vi "LINC Parser.vi"(8 "error in (no error)":errorcluster, 10 "command in":string) -> (0 "error out":errorcluster, 2 "command":string, 4 "command arguments":string[][](array[string]))   [LabVIEW 2018, in "STEPkgDriver_LINC.lvlib"]
doc: "Parses the string command to separate the command from the arguments. Provides syntax checking to ensure it follows the \"<CMD> WITH | TO<argument 1>,<argument 2>, etc\" syntax."
uses:
  STEPkgDriver_LINC.lvlib
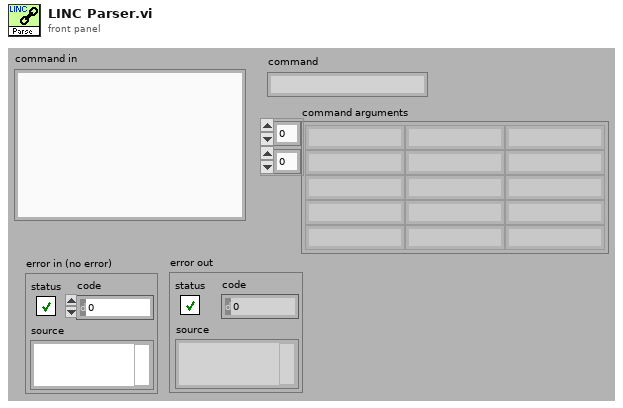
[diagram p1: front panel]
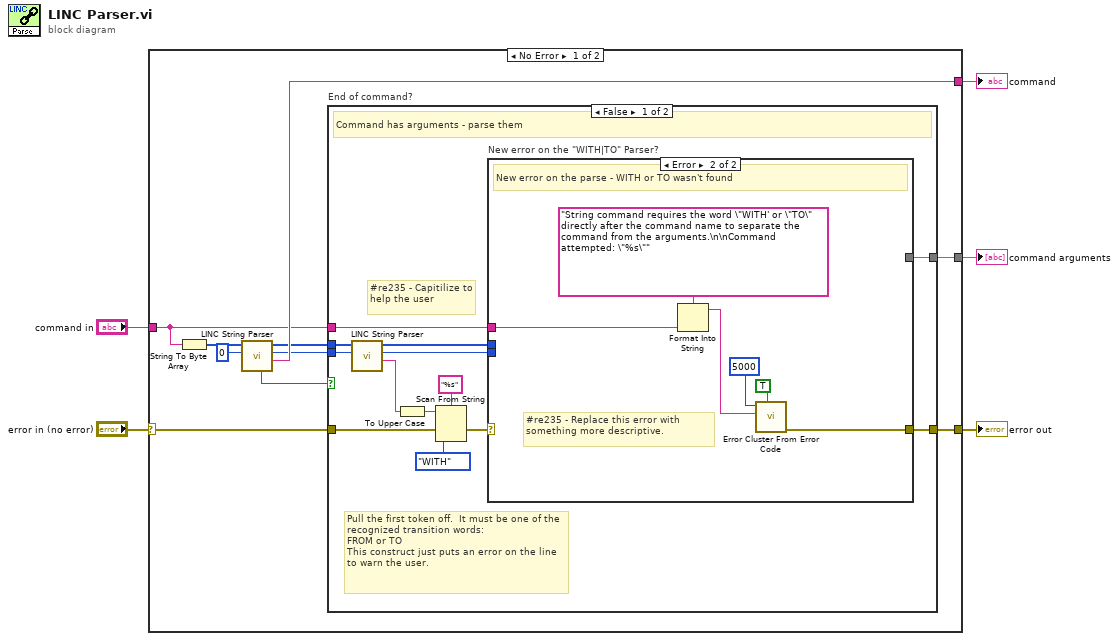
[diagram p0: block diagram]
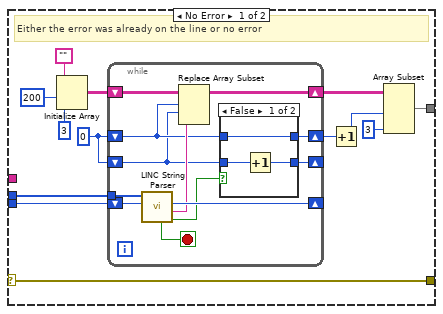
[diagram p2: hidden frame]
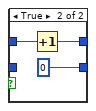
[diagram p3: hidden frame]
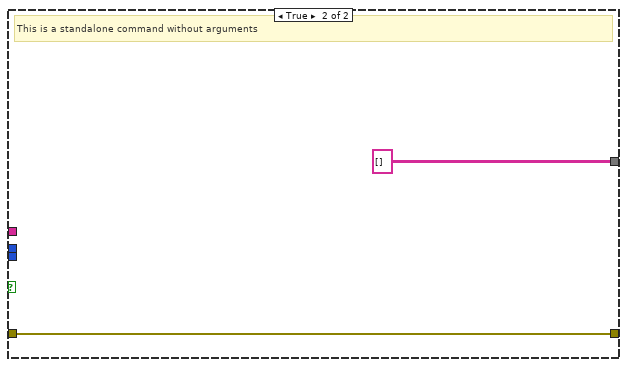
[diagram p4: hidden frame]
diagram:
  n1 = case shown="No Error" "error in (no error)" {
    selector: "error in (no error)" -> [w11 w68]
    tunnel: [w15 _] -> w5
    tunnel: [w14 w68] -> w4
    tunnel: [w13 _] -> w3
    tunnel: "command in" -> [w12 _]
    frame No Error {
      n2 = String To Byte Array(string=w12) -> (unsigned byte array=w10:u8[])
      n3 = call "LINC String Parser.vi"("index in"=0, "string in"=w10) -> ("string found"=w13:string, "index out"=w6:i32, "string out"=w7:u8[], "end"=w8:bool)  [unwired: 5 in, 1 out]
      n4 = case "End of command?" shown="False" w8 {
        tunnel: [w22 string[][] []] -> w15
        tunnel: w11 -> [w16 w67]
        tunnel: [w19 w67] -> w14
        tunnel: w7 -> [w26 _]
        tunnel: w6 -> [w25 _]
        tunnel: w12 -> [w18 _]
        frame False {
          # "#re235 - Capitilize to help the user"
          # "Pull the first token off.  It must be one of the recognized transition words:\nFROM or TO\nThis construct just puts an error on the line to warn the user."
          # "Command has arguments - parse them"
          n5 = call "LINC String Parser.vi"("index in"=w25, "string in"=w26) -> ("string found"=w21:string, "index out"=w24:i32, "string out"=w23:u8[])  [unwired: 5 in, 2 out]
          n6 = To Upper Case(1:w21) -> (0:w20:string)
          n7 = Scan From String(format string="%s", input string=w20, error in=w16, default 1=enum16{"WITH", "TO"}."WITH") -> (error out=w17:errorcluster)  [unwired: 2 in, 2 out]
          n8 = case "New error on the \"WITH|TO\" Parser?" shown="Error" w17 {
            selector: w17 -> [w29 _]
            tunnel: w24 -> [w41 _]
            tunnel: w23 -> [w40 _]
            tunnel: [w31 _] -> w22
            tunnel: [w29 w65] -> w19
            tunnel: w18 -> [_ w60]
            frame No Error {
              w35 = 0
              # "Either the error was already on the line or no error"
              n9 = Initialize Array("", 200, 3 ("dimension size")) -> (w36:string[][])
              n10 = while {
                shift-right: [w51] -> _
                shift-left: w41 -> [w52]
                tunnel: w40 -> [w53]
                shift-right: [w42] -> w34
                shift-left: w36 -> [w50]
                shift-right: [w44] -> w33
                shift-left: w35 -> [w48]
                shift-right: [w43] -> _
                shift-left: w35 -> [w47]
                stop <- w45 stop-if-true
                n11 = call "LINC String Parser.vi"("index in"=w52, "string in"=w53) -> ("comma found"=w46:bool, "string found"=w49:string, "index out"=w51:i32, "end"=w45:bool)  [unwired: 5 in, 1 out]
                n12 = Replace Array Subset(array=w50, new element=w49, index (row)=w48, index (col)=w47) -> (w42:string[][])
                n13 = case shown="False" w46 {
                  tunnel: w48 -> [w56 w59]
                  tunnel: w47 -> [w55 _]
                  tunnel: [w56 w58] -> w44
                  tunnel: [w54 0] -> w43
                  frame False {
                    n14 = Increment(x=w55) -> (x+1=w54:i32)
                  }
                  frame True {
                    n15 = Increment(x=w59) -> (x+1=w58:i32)
                  }
                }
              }
              n16 = Increment(x=w33) -> (x+1=w30:i32)
              n17 = Array Subset(array=w34, length (row)=w30, length (col)=3 ("length")) -> (w31:string[][])  [unwired: 2 in]
            }
            frame Error {
              # "#re235 - Replace this error with something more descriptive."
              # "New error on the parse - WITH or TO wasn't found"
              n18 = Format Into String(format string="String command requires the word \"WITH' or \"TO\" directly after the command name to separate the command from the arguments.\n\nCommand attempted: \"%s\"" ("error message (\"\")"), w60) -> (resulting string=w61:string)  [unwired: 2 in, 1 out]
              n19 = call <vilib>:"Error Cluster From Error Code.vi"("show call chain? (False)"=TRUE, "error message (\"\")"=w61, "error code (0)"=5000) -> ("error out"=w65:errorcluster)  [unwired: 6 in]
            }
          }
        }
        frame True {
          # "This is a standalone command without arguments"
        }
      }
    }
    frame Error {
    }
  }
  "command arguments" <- w5
  "command" <- w3
  "error out" <- w4
